vi "HFRR ADV v037 new software.vi"() -> ()   [LabVIEW 2025] (continued)
        n1886 = case shown="True" w2900 {
          frame False {
          }
          frame True {
            n1887 = local write "stopT"(FALSE) -> ()
          }
        }
      }
      frame True {
        "stopT" <- TRUE
      }
    }
    n1888 = case shown="False" w2210 {
      frame False {
      }
      frame True {
      }
    }
    n1889 = case shown="True" w2202 {
      frame False {
        n1890 = property on="Password 2" class="Str"("Visible"=FALSE) -> ()  [unwired: 2 in, 2 out]
        n1891 = local write "Password 2"("" ("Password")) -> ()
      }
      frame True {
        n1892 = property on="Password 2" class="Str"("Visible"=TRUE) -> ()  [unwired: 2 in, 2 out]
        n1893 = Equal?(x="Password 2", y="HFRR1234") -> (x = y?=w2225:bool)
        n1894 = case shown="True" w2225 {
          tunnel: "Password 2" -> [w2228 _]
          frame False {
            n1895 = String Length(string=w2228) -> (length=w2229:i32)
            n1896 = Greater Than 0?(x=w2229) -> (x > 0?=w2227:bool)
            n1897 = case shown="False" w2227 {
              frame False {
                n1898 = property on="Password 2" class="Str"("Caption.Text"="Password (Advance Setting)") -> ()  [unwired: 2 in, 2 out]
              }
              frame True {
                n1899 = property on="Password 2" class="Str"("Caption.Text"="Incorrect Password!") -> ()  [unwired: 2 in, 2 out]
              }
            }
          }
          frame True {
            n1900 = local write "EDIT 2"(FALSE ("EDIT 2")) -> ()
            n1901 = local write "Password 2"("" ("Password")) -> ()
            n1902 = local write "Main Tab"(T2."Advance" ("Main Tab")) -> ()
            n1903 = local write "Main Dashboard Buttons"(T1."Advance" ("Main Dashboard Buttons")) -> ()
          }
        }
      }
    }
    n1904 = case shown="True" "Prog Uno" {
      frame False {
      }
      frame True {
        n1905 = stacked-sequence {
          frame #0 {
            n1906 = Delete(path (use dialog)=path "C:/LAB-IQ-NXT/UNOCOMPILE.bat" ("working directory")) -> ()  [unwired: 4 in, 3 out]
          }
          frame #1 {
            n1907 = local read "Com Port 1"() -> (w2667:refnum<visa-resource-name>)
            n1908 = Concatenate Strings("cmd.exe /c \"mode " ("command line"), w2667, ":1200,n,8,1\"\n" ("command line")) -> (w2672:string)
            n1909 = Concatenate Strings(w2672, "CD\\\nCD WinDucom\navrdude -C avrdude.conf -v -patmega328p -carduino -P" ("command line"), w2667, " -b115200 -D -Uflash:w:UNO_V20.hex:i\n" ("command line"), "\r") -> (w2674:string)
            "STR" <- w2674
            n1910 = call <vilib>:"Write Characters To File.vi"("append to file? (new file:F)"=FALSE, "character string"=w2674, "file path (dialog if empty)"=path "C:/LAB-IQ/UNOCOMPILE.bat" ("working directory")) -> ()  [unwired: 2 in, 1 out]
          }
          frame #2 {
            n1911 = disable-structure shown="Disabled" {
              frame Disabled {
                w2678 = "cmd.exe  /c \"C:\\LAB-IQ-NXT\\UNOCOMPILE.bat\"" ("string")
                n1912 = local write "Prog Uno"(FALSE ("run minimized? (F)")) -> ()
                n1913 = call <vilib>:"System Exec.vi"("expected output size  (4096)"=u32 65535, "run minimized? (F)"=FALSE, "wait until completion? (T)"=TRUE ("run minimized? (F)"), "working directory"=path "C:/LAB-IQ-NXT", "standard input"=w2678, "command line"=w2678) -> ("error out"=w2677:errorcluster, "standard output"=→"String 42":string)  [unwired: 2 in, 2 out]
                "error out 3" <- w2677
                n1914 = flat-sequence {
                  tunnel: w2677 -> [_]
                  frame #0 {
                  }
                }
              }
              frame Enabled {
              }
            }
          }
        }
      }
    }
    n1915 = case shown="\"ISO 12156\"" "TEST STANDARD" {
      frame "ASTM D6079", Default {
        w2647 = 50.0 ("Hz")
        w2648 = 53.0 ("Set Rh")
        w2650 = 1.0 ("Set Strk")
        w2649 = 60.0 ("Set Temp")
        # "astm hide"
        n1916 = local write "NORMAL LOAD"(200.0 ("NORMAL LOAD")) -> ()
        n1917 = local write "Set Strk"(w2650) -> ()
        n1918 = local write "Set Hz"(w2647) -> ()
        n1919 = local write "Set Temp"(w2649) -> ()
        n1920 = local write "Set Rh"(w2648) -> ()
        n1921 = local write "test time"(75.0 ("test time")) -> ()
        n1922 = local write "Set Stroke:"(w2650) -> ()
        n1923 = local write "Set Humidity:"(w2648) -> ()
        n1924 = local write "Set Frequency:"(w2647) -> ()
        n1925 = local write "Set Temperature:"(w2649) -> ()
        "Test Standard" <- "ASTM D6079" ("Test Standard 2")
      }
      frame "ISO 12156" {
        n1926 = local write "Set Strk"(1.0 ("Set Strk")) -> ()
        n1927 = local write "NORMAL LOAD"(200.0 ("NORMAL LOAD")) -> ()
        n1928 = local write "Set Temp"(60.0 ("Set Temp")) -> ()
        n1929 = local write "test time"(75.0 ("test time")) -> ()
        n1930 = local write "Set Hz"(50.0 ("Hz")) -> ()
        n1931 = local write "Set Rh"(53.0 ("Set Rh")) -> ()
      }
      frame "CEC F-096-A-06" {
        n1932 = local write "Set Strk"(1.0 ("Set Strk")) -> ()
        n1933 = local write "NORMAL LOAD"(200.0 ("NORMAL LOAD")) -> ()
        n1934 = local write "Set Temp"(60.0 ("Set Temp")) -> ()
        n1935 = local write "test time"(75.0 ("test time")) -> ()
        n1936 = local write "Set Hz"(50.0 ("Hz")) -> ()
        n1937 = local write "Set Rh"(53.0 ("Set Rh")) -> ()
      }
      frame "Custom" {
      }
    }
    n1938 = Or(x=w2200, y=w2198) -> (x .or. y?=w2199:bool)
    n1939 = case shown="\"About\"" w2197 {
      tunnel: [T28."Acquire" ("Main Tab") T28."Compare Files" ("Main Tab") T28."About" ("Main Tab")] -> w2208
      frame "Acquire", Default {
      }
      frame "Compare Files" {
      }
      frame "About" {
      }
    }
    n1940 = Or(x=w2203, y="OPEN") -> (x .or. y?=w2204:bool)
    n1941 = case shown="True" w2204 {
      tunnel: w2203 -> [_ w2236]
      frame False {
      }
      frame True {
        n1942 = stacked-sequence {
          tunnel: w2236 -> [_ w2303 _ _]
          frame #0 {
            w2252 = "  " ("String 6")
            n1943 = local write "OPEN"(FALSE ("open")) -> ()
            n1944 = local read "string1 2"() -> (w2240:string)
            n1945 = local read "string1 3"() -> (w2239:string)
            n1946 = local read "string1 4"() -> (w2238:string)
            n1947 = property on="OPEN" class="Bool (strict)"("Visible"=FALSE) -> ()  [unwired: 2 in, 2 out]
            n1948 = local write "String 6"(w2252) -> ()
            n1949 = local write "String 7"(w2252) -> ()
            n1950 = local write "String 8"(w2252) -> ()
            n1951 = local write "String 12"(w2252) -> ()
            n1952 = local read "OK Button 16"() -> (w2237:bool)
            n1953 = String To Path(string=w2240) -> (path=w2248:path)
            n1954 = String To Path(string=w2239) -> (path=w2247:path)
            n1955 = String To Path(string=w2238) -> (path=w2246:path)
            n1956 = case shown="True" w2237 {
              tunnel: [w2253 w2254] -> w2241
              frame False {
                n1957 = local read "string1"() -> (w2253:string)
              }
              frame True {
                n1958 = local read "String Indicator 4"() -> (w2254:string)
              }
            }
            n1959 = Open/Create/Replace File "Open File"(file path (use dialog)=w2248) -> (refnum out=w2244:refnum<file>)  [unwired: 5 in, 2 out]
            n1960 = Open/Create/Replace File "Open File"(file path (use dialog)=w2247) -> (refnum out=w2243:refnum<file>)  [unwired: 5 in, 2 out]
            n1961 = Open/Create/Replace File "Open File"(file path (use dialog)=w2246) -> (refnum out=w2242:refnum<file>)  [unwired: 5 in, 2 out]
            n1962 = while {
              tunnel: w2244 -> [w2266]
              i -> [w2262]
              stop <- w2261 continue-if-true
              (unwired) TRUE ("line mode (F)")
              n1963 = Read from Text File "Read File"(file (use dialog)=w2266) -> (text=w2263:string)  [unwired: 3 in, 3 out]
              n1964 = local write "Numeric 11"(w2262) -> ()
              n1965 = String Length(string=w2263) -> (length=w2265:i32)
              n1966 = Greater?(x=w2265, y=1) -> (0:w2261:bool)
            }
            n1967 = while {
              tunnel: w2243 -> [w2272]
              i -> [w2268]
              stop <- w2267 continue-if-true
              (unwired) TRUE ("line mode (F)")
              n1968 = Read from Text File "Read File"(file (use dialog)=w2272) -> (text=w2269:string)  [unwired: 3 in, 3 out]
              n1969 = local write "Numeric 12"(w2268) -> ()
              n1970 = String Length(string=w2269) -> (length=w2271:i32)
              n1971 = Greater?(x=w2271, y=1) -> (0:w2267:bool)
            }
            n1972 = while {
              tunnel: w2242 -> [w2278]
              i -> [w2274]
              stop <- w2273 continue-if-true
              (unwired) TRUE ("line mode (F)")
              n1973 = Read from Text File "Read File"(file (use dialog)=w2278) -> (text=w2275:string)  [unwired: 3 in, 3 out]
              n1974 = local write "Numeric 13"(w2274) -> ()
              n1975 = String Length(string=w2275) -> (length=w2277:i32)
              n1976 = Greater?(x=w2277, y=1) -> (0:w2273:bool)
            }
            n1977 = String To Path(string=w2241) -> (path=w2249:path)
            n1978 = Open/Create/Replace File "Open File"(file path (use dialog)=w2249) -> (refnum out=w2245:refnum<file>)  [unwired: 5 in, 2 out]
            n1979 = while {
              tunnel: w2245 -> [w2260]
              i -> [w2256]
              stop <- w2255 continue-if-true
              (unwired) TRUE ("line mode (F)")
              n1980 = Read from Text File "Read File"(file (use dialog)=w2260) -> (text=w2257:string)  [unwired: 3 in, 3 out]
              n1981 = local write "Numeric 8"(w2256) -> ()
              n1982 = String Length(string=w2257) -> (length=w2259:i32)
              n1983 = Greater?(x=w2259, y=1) -> (0:w2255:bool)
            }
          }
          frame #1 {
            w2430 = FALSE ("ACTUAL   MERGE")
            # "Sample Temp"
            # "ECR"
            # "COF"
            # "Time\nCOF\nFF\nTemp"
            n1984 = case shown="True" w2303 {
              tunnel: [w2450 w2451] -> w2304
              frame False {
                n1985 = local read "string1"() -> (w2450:string)
              }
              frame True {
                n1986 = local read "String Indicator 4"() -> (w2451:string)
              }
            }
            n1987 = local read "string1 3"() -> (w2348:string)
            n1988 = String To Path(string=w2304) -> (path=w2435:path)
            n1989 = String To Path(string=w2348) -> (path=w2446:path)
            n1990 = local read "Numeric 12"() -> (w2432:i32)
            n1991 = local read "Numeric 8"() -> (w2434:i32)
            n1992 = local read "string1 2"() -> (w2349:string)
            n1993 = local read "string1 4"() -> (w2347:string)
            n1994 = Open/Create/Replace File "Open File"(file path (use dialog)=w2435) -> (refnum out=w2449:refnum<file>, error out=w2448:errorcluster)  [unwired: 5 in, 1 out]
            n1995 = Open/Create/Replace File "Open File"(file path (use dialog)=w2446) -> (refnum out=w2442:refnum<file>, error out=w2443:errorcluster)  [unwired: 5 in, 1 out]
            n1996 = for {
              N: w2434 -> [_]
              tunnel: w2449 -> [w2597]
              tunnel: w2448 -> [w2596]
              tunnel: [w2586] -> w2361 mode=indexing
              tunnel: [w2584] -> w2418 mode=indexing
              tunnel: [w2585] -> w2413 mode=indexing
              tunnel: w2430 -> [_]
              tunnel: [w2578] -> w2415 mode=indexing
              tunnel: [w2574] -> w2384 mode=indexing
              tunnel: [w2570] -> w2359 mode=indexing
              tunnel: [w2566] -> w2340 mode=indexing
              tunnel: [w2561] -> w2300 mode=indexing
              (unwired) TRUE ("line mode (F)")
              # "freq"
              # "Stroke"
              # "Time"
              # "CoF"
              # "Humidity"
              # "Temp"
              # "Air Temp"
              # "ECR"
              n1997 = Read from Text File "Read File"(file (use dialog)=w2597, error in=w2596) -> (text=w2562:string)  [unwired: 2 in, 3 out]
              n1998 = local write "String 6"(w2562) -> ()
              n1999 = String Subset(string=w2562, offset (0)=0, length (rest)=14 ("length (rest)")) -> (substring=w2590:string)
              n2000 = String Subset(string=w2562, offset (0)=35, length (rest)=9 ("length (rest)")) -> (substring=w2587:string)
              n2001 = String Subset(string=w2562, offset (0)=15, length (rest)=9 ("length (rest)")) -> (substring=w2593:string)
              n2002 = Fract/Exp String To Number(string=w2590) -> (number=w2586:dbl)  [unwired: 3 in, 1 out]
              n2003 = Fract/Exp String To Number(string=w2587) -> (number=w2585:dbl)  [unwired: 3 in, 1 out]
              n2004 = Fract/Exp String To Number(string=w2593) -> (number=w2584:dbl)  [unwired: 3 in, 1 out]
              n2005 = String Subset(string=w2562, offset (0)=85, length (rest)=9 ("length (rest)")) -> (substring=w2563:string)
              n2006 = String Subset(string=w2562, offset (0)=25, length (rest)=9 ("length (rest)")) -> (substring=w2569:string)
              n2007 = String Subset(string=w2562, offset (0)=55, length (rest)=9 ("length (rest)")) -> (substring=w2571:string)
              n2008 = String Subset(string=w2562, offset (0)=45, length (rest)=9 ("length (rest)")) -> (substring=w2577:string)
              n2009 = String Subset(string=w2562, offset (0)=65, length (rest)=9 ("length (rest)")) -> (substring=w2583:string)
              n2010 = Fract/Exp String To Number(string=w2569) -> (number=w2566:dbl)  [unwired: 3 in, 1 out]
              n2011 = Fract/Exp String To Number(string=w2563) -> (number=w2561:dbl)  [unwired: 3 in, 1 out]
              n2012 = Fract/Exp String To Number(string=w2571) -> (number=w2570:dbl)  [unwired: 3 in, 1 out]
              n2013 = Fract/Exp String To Number(string=w2577) -> (number=w2574:dbl)  [unwired: 3 in, 1 out]
              n2014 = Fract/Exp String To Number(string=w2583) -> (number=w2580:dbl)  [unwired: 3 in, 1 out]
              n2015 = Add(x=w2580, y=0.0) -> (x+y=w2578:dbl)
            }
            n2016 = for {
              N: w2432 -> [_]
              tunnel: w2443 -> [w2523]
              tunnel: w2442 -> [w2522]
              tunnel: [w2512] -> w2401 mode=indexing
              tunnel: [w2510] -> w2399 mode=indexing
              tunnel: [w2511] -> w2395 mode=indexing
              tunnel: w2430 -> [_]
              tunnel: [w2504] -> w2397 mode=indexing
              tunnel: [w2500] -> w2379 mode=indexing
              tunnel: [w2496] -> w2355 mode=indexing
              tunnel: [w2493] -> w2336 mode=indexing
              tunnel: [w2489] -> w2295 mode=indexing
              (unwired) 9 ("length (rest)")
              (unwired) 9 ("length (rest)")
              (unwired) TRUE ("line mode (F)")
              n2017 = Read from Text File "Read File"(file (use dialog)=w2522, error in=w2523) -> (text=w2490:string)  [unwired: 2 in, 3 out]
              n2018 = local write "String 8"(w2490) -> ()
              n2019 = String Subset(string=w2490, offset (0)=85) -> (substring=w2492:string)  [unwired: 1 in]
              n2020 = String Subset(string=w2490, offset (0)=35, length (rest)=9 ("length (rest)")) -> (substring=w2513:string)
              n2021 = String Subset(string=w2490, offset (0)=55, length (rest)=9 ("length (rest)")) -> (substring=w2498:string)
              n2022 = String Subset(string=w2490, offset (0)=25) -> (substring=w2494:string)  [unwired: 1 in]
              n2023 = String Subset(string=w2490, offset (0)=15, length (rest)=9 ("length (rest)")) -> (substring=w2519:string)
              n2024 = String Subset(string=w2490, offset (0)=0, length (rest)=14 ("length (rest)")) -> (substring=w2516:string)
              n2025 = String Subset(string=w2490, offset (0)=45, length (rest)=9 ("length (rest)")) -> (substring=w2503:string)
              n2026 = String Subset(string=w2490, offset (0)=65, length (rest)=9 ("length (rest)")) -> (substring=w2509:string)
              n2027 = Fract/Exp String To Number(string=w2492) -> (number=w2489:dbl)  [unwired: 3 in, 1 out]
              n2028 = Fract/Exp String To Number(string=w2513) -> (number=w2511:dbl)  [unwired: 3 in, 1 out]
              n2029 = Fract/Exp String To Number(string=w2498) -> (number=w2496:dbl)  [unwired: 3 in, 1 out]
              n2030 = Fract/Exp String To Number(string=w2494) -> (number=w2493:dbl)  [unwired: 3 in, 1 out]
              n2031 = Fract/Exp String To Number(string=w2519) -> (number=w2510:dbl)  [unwired: 3 in, 1 out]
              n2032 = Fract/Exp String To Number(string=w2516) -> (number=w2512:dbl)  [unwired: 3 in, 1 out]
              n2033 = Fract/Exp String To Number(string=w2503) -> (number=w2500:dbl)  [unwired: 3 in, 1 out]
              n2034 = Fract/Exp String To Number(string=w2509) -> (number=w2506:dbl)  [unwired: 3 in, 1 out]
              n2035 = Add(x=w2506, y=0.0) -> (x+y=w2504:dbl)
            }
            n2036 = String To Path(string=w2349) -> (path=w2447:path)
            n2037 = String To Path(string=w2347) -> (path=w2441:path)
            n2038 = local read "Numeric 11"() -> (w2431:i32)
            n2039 = local read "Numeric 13"() -> (w2433:i32)
            n2040 = Open/Create/Replace File "Open File"(file path (use dialog)=w2447) -> (refnum out=w2445:refnum<file>, error out=w2444:errorcluster)  [unwired: 5 in, 1 out]
            n2041 = Open/Create/Replace File "Open File"(file path (use dialog)=w2441) -> (refnum out=w2440:refnum<file>, error out=w2439:errorcluster)  [unwired: 5 in, 1 out]
            n2042 = for {
              N: w2431 -> [_]
              tunnel: w2445 -> [w2560]
              tunnel: w2444 -> [w2559]
              tunnel: [w2549] -> w2411 mode=indexing
              tunnel: [w2547] -> w2409 mode=indexing
              tunnel: [w2548] -> w2404 mode=indexing
              tunnel: w2430 -> [_]
              tunnel: [w2541] -> w2406 mode=indexing
              tunnel: [w2537] -> w2382 mode=indexing
              tunnel: [w2533] -> w2357 mode=indexing
              tunnel: [w2529] -> w2338 mode=indexing
              tunnel: [w2524] -> w2296 mode=indexing
              (unwired) TRUE ("line mode (F)")
              n2043 = Read from Text File "Read File"(file (use dialog)=w2560, error in=w2559) -> (text=w2525:string)  [unwired: 2 in, 3 out]
              n2044 = local write "String 7"(w2525) -> ()
              n2045 = String Subset(string=w2525, offset (0)=85, length (rest)=9 ("length (rest)")) -> (substring=w2528:string)
              n2046 = String Subset(string=w2525, offset (0)=35, length (rest)=9 ("length (rest)")) -> (substring=w2550:string)
              n2047 = String Subset(string=w2525, offset (0)=55, length (rest)=9 ("length (rest)")) -> (substring=w2536:string)
              n2048 = String Subset(string=w2525, offset (0)=25, length (rest)=9 ("length (rest)")) -> (substring=w2530:string)
              n2049 = String Subset(string=w2525, offset (0)=45, length (rest)=9 ("length (rest)")) -> (substring=w2538:string)
              n2050 = String Subset(string=w2525, offset (0)=0, length (rest)=14 ("length (rest)")) -> (substring=w2553:string)
              n2051 = String Subset(string=w2525, offset (0)=15, length (rest)=9 ("length (rest)")) -> (substring=w2556:string)
              n2052 = String Subset(string=w2525, offset (0)=65, length (rest)=9 ("length (rest)")) -> (substring=w2542:string)
              n2053 = Fract/Exp String To Number(string=w2528) -> (number=w2524:dbl)  [unwired: 3 in, 1 out]
              n2054 = Fract/Exp String To Number(string=w2550) -> (number=w2548:dbl)  [unwired: 3 in, 1 out]
              n2055 = Fract/Exp String To Number(string=w2536) -> (number=w2533:dbl)  [unwired: 3 in, 1 out]
              n2056 = Fract/Exp String To Number(string=w2530) -> (number=w2529:dbl)  [unwired: 3 in, 1 out]
              n2057 = Fract/Exp String To Number(string=w2538) -> (number=w2537:dbl)  [unwired: 3 in, 1 out]
              n2058 = Fract/Exp String To Number(string=w2553) -> (number=w2549:dbl)  [unwired: 3 in, 1 out]
              n2059 = Fract/Exp String To Number(string=w2556) -> (number=w2547:dbl)  [unwired: 3 in, 1 out]
              n2060 = Fract/Exp String To Number(string=w2542) -> (number=w2545:dbl)  [unwired: 3 in, 1 out]
              n2061 = Add(x=w2545, y=0.0) -> (x+y=w2541:dbl)
            }
            n2062 = for {
              N: w2433 -> [_]
              tunnel: w2440 -> [w2488]
              tunnel: w2439 -> [w2487]
              tunnel: [w2477] -> w2393 mode=indexing
              tunnel: [w2476] -> w2386 mode=indexing
              tunnel: w2430 -> [_]
              tunnel: [w2465] -> w2391 mode=indexing
              tunnel: [w2470] -> w2388 mode=indexing
              tunnel: [w2466] -> w2378 mode=indexing
              tunnel: [w2461] -> w2353 mode=indexing
              tunnel: [w2457] -> w2334 mode=indexing
              tunnel: [w2452] -> w2294 mode=indexing
              (unwired) 1.0 ("x")
              (unwired) TRUE ("line mode (F)")
              n2063 = Read from Text File "Read File"(file (use dialog)=w2488, error in=w2487) -> (text=w2453:string)  [unwired: 2 in, 3 out]
              n2064 = local write "String 12"(w2453) -> ()
              n2065 = String Subset(string=w2453, offset (0)=85, length (rest)=9 ("length (rest)")) -> (substring=w2455:string)
              n2066 = String Subset(string=w2453, offset (0)=35, length (rest)=9 ("length (rest)")) -> (substring=w2478:string)
              n2067 = String Subset(string=w2453, offset (0)=55, length (rest)=9 ("length (rest)")) -> (substring=w2463:string)
              n2068 = String Subset(string=w2453, offset (0)=25, length (rest)=9 ("length (rest)")) -> (substring=w2459:string)
              n2069 = String Subset(string=w2453, offset (0)=45, length (rest)=9 ("length (rest)")) -> (substring=w2468:string)
              n2070 = String Subset(string=w2453, offset (0)=15, length (rest)=9 ("length (rest)")) -> (substring=w2484:string)
              n2071 = String Subset(string=w2453, offset (0)=0, length (rest)=14 ("length (rest)")) -> (substring=w2481:string)
              n2072 = String Subset(string=w2453, offset (0)=65, length (rest)=9 ("length (rest)")) -> (substring=w2471:string)
              n2073 = Fract/Exp String To Number(string=w2455) -> (number=w2452:dbl)  [unwired: 3 in, 1 out]
              n2074 = Fract/Exp String To Number(string=w2478) -> (number=w2476:dbl)  [unwired: 3 in, 1 out]
              n2075 = Fract/Exp String To Number(string=w2463) -> (number=w2461:dbl)  [unwired: 3 in, 1 out]
              n2076 = Fract/Exp String To Number(string=w2459) -> (number=w2457:dbl)  [unwired: 3 in, 1 out]
              n2077 = Fract/Exp String To Number(string=w2468) -> (number=w2466:dbl)  [unwired: 3 in, 1 out]
              n2078 = Fract/Exp String To Number(string=w2484) -> (number=w2465:dbl)  [unwired: 3 in, 1 out]
              n2079 = Fract/Exp String To Number(string=w2481) -> (number=w2477:dbl)  [unwired: 3 in, 1 out]
              n2080 = Fract/Exp String To Number(string=w2471) -> (number=w2474:dbl)  [unwired: 3 in, 1 out]
              n2081 = Add(x=w2474, y=0.0) -> (x+y=w2470:dbl)
            }
            n2082 = Delete From Array(array=w2336, index=0) -> (array with subset deleted=w2309:dbl[])  [unwired: 1 in, 1 out]
            n2083 = Delete From Array(array=w2399, index=0) -> (array with subset deleted=w2372:dbl[])  [unwired: 1 in, 1 out]
            n2084 = Delete From Array(array=w2379, index=0) -> (array with subset deleted=w2367:dbl[])  [unwired: 1 in, 1 out]
            n2085 = Delete From Array(array=w2397, index=0) -> (array with subset deleted=w2398:dbl[])  [unwired: 1 in, 1 out]
            n2086 = call-poly <vilib>:"Mean.vi"("X"=w2309) -> ("mean"=→"КОФ2 4":dbl)  [unwired: 1 out]
            n2087 = call-poly <vilib>:"Mean.vi"("X"=w2372) -> ("mean"=→"КОФ3":dbl)  [unwired: 1 out]
            n2088 = call-poly <vilib>:"Mean.vi"("X"=w2367) -> ("mean"=→"CP3":dbl)  [unwired: 1 out]
            n2089 = Delete From Array(array=w2361, index=0) -> (array with subset deleted=w2288:dbl[])  [unwired: 1 in, 1 out]
            n2090 = Delete From Array(array=w2300, index=0) -> (array with subset deleted=w2287:dbl[])  [unwired: 1 in, 1 out]
            n2091 = Delete From Array(array=w2340, index=0) -> (array with subset deleted=w2311:dbl[])  [unwired: 1 in, 1 out]
            n2092 = Delete From Array(array=w2418, index=0) -> (array with subset deleted=w2373:dbl[])  [unwired: 1 in, 1 out]
            n2093 = Delete From Array(array=w2384, index=0) -> (array with subset deleted=w2369:dbl[])  [unwired: 1 in, 1 out]
            "array w/ subset deleted" <- w2369
            n2094 = Delete From Array(array=w2415, index=0) -> (array with subset deleted=w2416:dbl[])  [unwired: 1 in, 1 out]
            n2095 = call-poly <vilib>:"Mean.vi"("X"=w2311) -> ("mean"=→"КОФ2 2":dbl)  [unwired: 1 out]
            n2096 = call-poly <vilib>:"Mean.vi"("X"=w2373) -> ("mean"=→"КОФ1":dbl)  [unwired: 1 out]
            n2097 = Bundle "Bundle"(w2288, w2287) -> (w2293:cluster{dbl[], dbl[]})  [unwired: 1 in]
            n2098 = Bundle "Bundle"(w2288, w2416) -> (w2280:cluster{dbl[], dbl[]})  [unwired: 1 in]
            n2099 = Delete From Array(array=w2295, index=0) -> (array with subset deleted=w2283:dbl[])  [unwired: 1 in, 1 out]
            n2100 = Delete From Array(array=w2296, index=0) -> (array with subset deleted=w2285:dbl[])  [unwired: 1 in, 1 out]
            n2101 = Delete From Array(array=w2406, index=0) -> (array with subset deleted=w2407:dbl[])  [unwired: 1 in, 1 out]
            n2102 = Delete From Array(array=w2294, index=0) -> (array with subset deleted=w2281:dbl[])  [unwired: 1 in, 1 out]
            n2103 = Delete From Array(array=w2388, index=0) -> (array with subset deleted=w2389:dbl[])  [unwired: 1 in, 1 out]
            n2104 = Delete From Array(array=w2413, index=0) -> (array with subset deleted=w2319:dbl[])  [unwired: 1 in, 1 out]
            n2105 = Delete From Array(array=w2359, index=0) -> (array with subset deleted=w2315:dbl[])  [unwired: 1 in, 1 out]
            n2106 = Delete From Array(array=w2395, index=0) -> (array with subset deleted=w2317:dbl[])  [unwired: 1 in, 1 out]
            n2107 = Delete From Array(array=w2355, index=0) -> (array with subset deleted=w2313:dbl[])  [unwired: 1 in, 1 out]
            n2108 = Delete From Array(array=w2404, index=0) -> (array with subset deleted=w2318:dbl[])  [unwired: 1 in, 1 out]
            n2109 = Delete From Array(array=w2357, index=0) -> (array with subset deleted=w2314:dbl[])  [unwired: 1 in, 1 out]
            n2110 = Delete From Array(array=w2338, index=0) -> (array with subset deleted=w2310:dbl[])  [unwired: 1 in, 1 out]
            n2111 = Delete From Array(array=w2382, index=0) -> (array with subset deleted=w2368:dbl[])  [unwired: 1 in, 1 out]
            n2112 = Delete From Array(array=w2409, index=0) -> (array with subset deleted=w2370:dbl[])  [unwired: 1 in, 1 out]
            n2113 = Delete From Array(array=w2386, index=0) -> (array with subset deleted=w2316:dbl[])  [unwired: 1 in, 1 out]
            n2114 = Delete From Array(array=w2353, index=0) -> (array with subset deleted=w2312:dbl[])  [unwired: 1 in, 1 out]
            n2115 = Delete From Array(array=w2334, index=0) -> (array with subset deleted=w2308:dbl[])  [unwired: 1 in, 1 out]
            n2116 = Delete From Array(array=w2378, index=0) -> (array with subset deleted=w2366:dbl[])  [unwired: 1 in, 1 out]
            n2117 = Delete From Array(array=w2391, index=0) -> (array with subset deleted=w2371:dbl[])  [unwired: 1 in, 1 out]
            n2118 = Delete From Array(array=w2401, index=0) -> (array with subset deleted=w2284:dbl[])  [unwired: 1 in, 1 out]
            n2119 = Delete From Array(array=w2411, index=0) -> (array with subset deleted=w2286:dbl[])  [unwired: 1 in, 1 out]
            n2120 = Delete From Array(array=w2393, index=0) -> (array with subset deleted=w2282:dbl[])  [unwired: 1 in, 1 out]
            n2121 = Bundle "Bundle"(w2288, w2319) -> (w2306:cluster{dbl[], dbl[]})  [unwired: 1 in]
            n2122 = Bundle "Bundle"(w2288, w2373) -> (w2307:cluster{dbl[], dbl[]})  [unwired: 1 in]
            n2123 = Bundle "Bundle"(w2319, w2315) -> (w2321:cluster{dbl[], dbl[]})  [unwired: 1 in]
            n2124 = Bundle "Bundle"(w2284, w2283) -> (w2291:cluster{dbl[], dbl[]})  [unwired: 1 in]
            n2125 = Bundle "Bundle"(w2317, w2313) -> (w2323:cluster{dbl[], dbl[]})  [unwired: 1 in]
            n2126 = Bundle "Bundle"(w2284, w2317) -> (w2427:cluster{dbl[], dbl[]})  [unwired: 1 in]
            n2127 = Bundle "Bundle"(w2284, w2313) -> (w2351:cluster{dbl[], dbl[]})  [unwired: 1 in]
            n2128 = Bundle "Bundle"(w2284, w2372) -> (w2437:cluster{dbl[], dbl[]})  [unwired: 1 in]
            n2129 = Bundle "Bundle"(w2284, w2367) -> (w2375:cluster{dbl[], dbl[]})  [unwired: 1 in]
            n2130 = Bundle "Bundle"(w2284, w2398) -> (w2422:cluster{dbl[], dbl[]})  [unwired: 1 in]
            n2131 = Bundle "Bundle"(w2318, w2314) -> (w2322:cluster{dbl[], dbl[]})  [unwired: 1 in]
            n2132 = Bundle "Bundle"(w2286, w2285) -> (w2292:cluster{dbl[], dbl[]})  [unwired: 1 in]
            n2133 = Bundle "Bundle"(w2286, w2318) -> (w2429:cluster{dbl[], dbl[]})  [unwired: 1 in]
            n2134 = Bundle "Bundle"(w2286, w2314) -> (w2352:cluster{dbl[], dbl[]})  [unwired: 1 in]
            n2135 = Bundle "Bundle"(w2286, w2368) -> (w2376:cluster{dbl[], dbl[]})  [unwired: 1 in]
            n2136 = Bundle "Bundle"(w2286, w2370) -> (w2438:cluster{dbl[], dbl[]})  [unwired: 1 in]
            n2137 = Bundle "Bundle"(w2286, w2407) -> (w2420:cluster{dbl[], dbl[]})  [unwired: 1 in]
            n2138 = Bundle "Bundle"(w2316, w2312) -> (w2324:cluster{dbl[], dbl[]})  [unwired: 1 in]
            n2139 = Bundle "Bundle"(w2282, w2281) -> (w2290:cluster{dbl[], dbl[]})  [unwired: 1 in]
            n2140 = Bundle "Bundle"(w2282, w2316) -> (w2428:cluster{dbl[], dbl[]})  [unwired: 1 in]
            n2141 = Bundle "Bundle"(w2282, w2312) -> (w2350:cluster{dbl[], dbl[]})  [unwired: 1 in]
            n2142 = Bundle "Bundle"(w2282, w2366) -> (w2374:cluster{dbl[], dbl[]})  [unwired: 1 in]
            n2143 = Bundle "Bundle"(w2282, w2371) -> (w2436:cluster{dbl[], dbl[]})  [unwired: 1 in]
            n2144 = Bundle "Bundle"(w2282, w2389) -> (w2421:cluster{dbl[], dbl[]})  [unwired: 1 in]
            n2145 = call-poly <vilib>:"Mean.vi"("X"=w2369) -> ("mean"=→"CP1":dbl)  [unwired: 1 out]
            n2146 = call-poly <vilib>:"Mean.vi"("X"=w2310) -> ("mean"=→"КОФ2 3":dbl)  [unwired: 1 out]
            n2147 = call-poly <vilib>:"Mean.vi"("X"=w2368) -> ("mean"=→"CP2":dbl)  [unwired: 1 out]
            n2148 = call-poly <vilib>:"Mean.vi"("X"=w2370) -> ("mean"=→"КОФ2":dbl)  [unwired: 1 out]
            n2149 = call-poly <vilib>:"Mean.vi"("X"=w2308) -> ("mean"=→"КОФ2 5":dbl)  [unwired: 1 out]
            n2150 = call-poly <vilib>:"Mean.vi"("X"=w2366) -> ("mean"=→"CP4":dbl)  [unwired: 1 out]
            n2151 = call-poly <vilib>:"Mean.vi"("X"=w2371) -> ("mean"=→"КОФ4":dbl)  [unwired: 1 out]
            n2152 = Bundle "Bundle"(w2288, w2315) -> (w2279:cluster{dbl[], dbl[]})  [unwired: 1 in]
            n2153 = Bundle "Bundle"(w2288, w2369) -> (w2302:cluster{dbl[], dbl[]})  [unwired: 1 in]
            n2154 = Build Array "Build Array"(w2279, w2302) -> (w2305:cluster{dbl[], dbl[]}[])
            "XY Graph 17" <- w2305
            n2155 = Build Array "Build Array"(w2293, w2292, w2291, w2290) -> (→"Frequency ( Hz )":cluster{dbl[], dbl[]}[])
            n2156 = Build Array "Build Array"(w2321, w2322, w2323, w2324) -> (→"Air Temp ( °C ) vs Humidity ( % RH )":cluster{dbl[], dbl[]}[])
            n2157 = Build Array "Build Array"(w2306, w2429, w2427, w2428) -> (→"Air Temperature  ( °C )":cluster{dbl[], dbl[]}[])
            n2158 = Build Array "Build Array"(w2279, w2352, w2351, w2350) -> (→"Humidity ( %RH )":cluster{dbl[], dbl[]}[])
            n2159 = Build Array "Build Array"(w2307, w2438, w2437, w2436) -> (→"Coefficient Of Friction":cluster{dbl[], dbl[]}[])
            n2160 = Build Array "Build Array"(w2302, w2376, w2375, w2374) -> (→"Sample Temperature ( °C )":cluster{dbl[], dbl[]}[])
            n2161 = Build Array "Build Array"(w2280, w2420, w2422, w2421) -> (→"XY Graph 13":cluster{dbl[], dbl[]}[])
            n2162 = Bundle "Bundle"(w2288, w2311) -> (w2333:cluster{dbl[], dbl[]})  [unwired: 1 in]
            n2163 = Bundle "Bundle"(w2284, w2309) -> (w2331:cluster{dbl[], dbl[]})  [unwired: 1 in]
            n2164 = Bundle "Bundle"(w2286, w2310) -> (w2332:cluster{dbl[], dbl[]})  [unwired: 1 in]
            n2165 = Bundle "Bundle"(w2282, w2308) -> (w2330:cluster{dbl[], dbl[]})  [unwired: 1 in]
            n2166 = Build Array "Build Array"(w2333, w2332, w2331, w2330) -> (→"Stroke ( mm )":cluster{dbl[], dbl[]}[])
            n2167 = local write "XY Graph 16"(w2305) -> ()
          }
          frame #2 {
          }
          frame #3 {
            n2168 = local write "Numeric 8"(0 ("Numeric 8")) -> ()
            n2169 = local write "Numeric 11"(0 ("Numeric 11")) -> ()
            n2170 = local write "Numeric 12"(0 ("Numeric 12")) -> ()
            n2171 = local write "Numeric 13"(0 ("Numeric 13")) -> ()
            n2172 = property on="OPEN" class="Bool (strict)"("Visible"=TRUE) -> ()  [unwired: 2 in, 2 out]
            n2173 = local read "String Control 2"() -> (w2605:string)
            n2174 = local read "String Control 4"() -> (w2604:string)
            n2175 = local read "String Control 6"() -> (w2603:string)
            n2176 = local read "String Control 8"() -> (w2602:string)
            n2177 = Match Pattern(string=w2605, regular expression="Samples / cycle :- ") -> (after substring=w2619:string)  [unwired: 1 in, 3 out]
            n2178 = Match Pattern(string=w2605, regular expression="Frequency :- ") -> (after substring=w2638:string)  [unwired: 1 in, 3 out]
            n2179 = Match Pattern(string=w2604, regular expression="Samples / cycle :- ") -> (after substring=w2615:string)  [unwired: 1 in, 3 out]
            n2180 = Match Pattern(string=w2604, regular expression="Frequency :- ") -> (after substring=w2633:string)  [unwired: 1 in, 3 out]
            n2181 = Match Pattern(string=w2603, regular expression="Samples / cycle :- ") -> (after substring=w2611:string)  [unwired: 1 in, 3 out]
            n2182 = Match Pattern(string=w2603, regular expression="Frequency :- ") -> (after substring=w2628:string)  [unwired: 1 in, 3 out]
            n2183 = Match Pattern(string=w2602, regular expression="Samples / cycle :- ") -> (after substring=w2607:string)  [unwired: 1 in, 3 out]
            n2184 = Match Pattern(string=w2602, regular expression="Frequency :- ") -> (after substring=w2623:string)  [unwired: 1 in, 3 out]
            n2185 = String Subset(string=w2619, length (rest)=6 ("length (rest)")) -> (substring=w2621:string)  [unwired: 1 in]
            n2186 = String Subset(string=w2638, length (rest)=9 ("length (rest)")) -> (substring=w2640:string)  [unwired: 1 in]
            n2187 = String Subset(string=w2615, length (rest)=6 ("length (rest)")) -> (substring=w2617:string)  [unwired: 1 in]
            n2188 = String Subset(string=w2633, length (rest)=9 ("length (rest)")) -> (substring=w2635:string)  [unwired: 1 in]
            n2189 = String Subset(string=w2611, length (rest)=6 ("length (rest)")) -> (substring=w2613:string)  [unwired: 1 in]
            n2190 = String Subset(string=w2628, length (rest)=9 ("length (rest)")) -> (substring=w2630:string)  [unwired: 1 in]
            n2191 = String Subset(string=w2607, length (rest)=6 ("length (rest)")) -> (substring=w2609:string)  [unwired: 1 in]
            n2192 = String Subset(string=w2623, length (rest)=9 ("length (rest)")) -> (substring=w2625:string)  [unwired: 1 in]
            n2193 = Fract/Exp String To Number(string=w2621) -> (number=w2601:dbl)  [unwired: 3 in, 1 out]
            n2194 = Fract/Exp String To Number(string=w2640) -> (number=w2641:dbl)  [unwired: 3 in, 1 out]
            n2195 = Fract/Exp String To Number(string=w2617) -> (number=w2600:dbl)  [unwired: 3 in, 1 out]
            n2196 = Fract/Exp String To Number(string=w2635) -> (number=w2636:dbl)  [unwired: 3 in, 1 out]
            n2197 = Fract/Exp String To Number(string=w2613) -> (number=w2599:dbl)  [unwired: 3 in, 1 out]
            n2198 = Fract/Exp String To Number(string=w2630) -> (number=w2631:dbl)  [unwired: 3 in, 1 out]
            n2199 = Fract/Exp String To Number(string=w2609) -> (number=w2598:dbl)  [unwired: 3 in, 1 out]
            n2200 = Fract/Exp String To Number(string=w2625) -> (number=w2626:dbl)  [unwired: 3 in, 1 out]
            n2201 = local write "sample1"(w2601) -> ()
            n2202 = local write "freq1"(w2641) -> ()
            n2203 = local write "sample2"(w2600) -> ()
            n2204 = local write "freq2"(w2636) -> ()
            n2205 = local write "sample3"(w2599) -> ()
            n2206 = local write "freq3"(w2631) -> ()
            n2207 = local write "sample4"(w2598) -> ()
            n2208 = local write "freq 4"(w2626) -> ()
          }
        }
      }
    }
    n2209 = case shown="True" w2199 {
      selector: w2199 -> [_ w2218]
      frame False {
      }
      frame True {
        n2210 = Not(x=w2218) -> (.not. x?=w2214:bool)
        n2211 = local write "service 3"(w2214) -> ()
        n2212 = local write "OPEN 6"(w2214) -> ()
        n2213 = call <vilib>:"System Exec.vi"("wait until completion? (T)"=TRUE, "command line"="C:\\LAB-IQ\\Scar View.exe") -> ("error out"=→"error out 5":errorcluster)  [unwired: 6 in, 3 out]
      }
    }
    n2214 = case shown="\"Acquire\", Default" w2208 {
      frame "Acquire", Default {
        # "Elapsed time\ncof\nstroke\nAir temp\nTemp\nHumidity"
        n2215 = disable-structure shown="Disabled" {
          frame Disabled {
            n2216 = local read "Flag"() -> (w2917:dbl)
            n2217 = local read "RUN"() -> (w2914:bool)
            n2218 = Not(x=w2914) -> (.not. x?=w2913:bool)
            n2219 = Equal?(x=w2917, y=10.0) -> (x = y?=w2915:bool)
            n2220 = And(x=w2915, y=w2913) -> (x .and. y?=w2912:bool)
            n2221 = case shown="True" w2912 {
              frame False {
              }
              frame True {
                w2918 = FALSE ("Heater Button")
                n2222 = local write "Humidity"(w2918) -> ()
                n2223 = local write "Heater Button"(w2918) -> ()
              }
            }
          }
          frame Enabled {
          }
        }
        n2224 = disable-structure shown="Disabled" {
          frame Disabled {
            n2225 = case shown="True" {
              selector: _ -> [_ _]
              frame False {
              }
              frame True {
                w2967 = TRUE ("Heater")
                n2226 = local write "Humidity"(w2967) -> ()
                n2227 = local write "Heater Button"(w2967) -> ()
                n2228 = local read "TEST STANDARD"() -> (w2970:T3)
                n2229 = local read "TEST STANDARD"() -> (w2965:T3)
                n2230 = Equal?(x=w2970, y=enum16{"ASTM D6079", "ISO 12156", "Custom"}."ISO 12156" ("Test Standard")) -> (x = y?=w2968:bool)
                n2231 = Equal?(x=w2965, y=enum16{"ASTM D6079", "ISO 12156", "Custom"}."ASTM D6079" ("Test Standard")) -> (x = y?=w2964:bool)
                n2232 = case shown="True" w2968 {
                  frame False {
                  }
                  frame True {
                    n2233 = local write "airtempflg"(FALSE ("airtempflg")) -> ()
                    n2234 = local write item#-1(TRUE ("Heater")) -> ()
                  }
                }
                n2235 = case shown="True" w2964 {
                  frame False {
                  }
                  frame True {
                    n2236 = local write "airtempflg"(TRUE ("airtempflg")) -> ()
                    n2237 = local write item#-1(FALSE ("Heater")) -> ()
                  }
                }
              }
            }
          }
          frame Enabled {
          }
        }
        n2238 = stacked-sequence {
          frame #0 {
            n2239 = case shown="True" "RST FF" {
              frame False {
              }
              frame True {
                w2984 = 0.0 ("X Scale.Range:Maximum")
                n2240 = property on="Frictional Force ( N )" class="WFChart (strict)"("XScale.Maximum"=600.0 ("X Scale.Range:Maximum"), "XScale.Minimum"=w2984, "YScale.Maximum"=10.0 ("Y Scale.Range:Maximum"), "YScale.Minimum"=w2984) -> ()  [unwired: 2 in, 2 out]
              }
            }
          }
          frame #1 {
            n2241 = case shown="True" "RST TEMP" {
              frame False {
              }
              frame True {
                n2242 = property on="Temperature ( Deg C )" class="WFChart (strict)"("XScale.Minimum"=0.0 ("X Scale.Range:Minimum"), "XScale.Maximum"=600.0 ("X Scale.Range:Maximum"), "YScale.Minimum"=0.0 ("Y Scale.Range:Minimum"), "YScale.Maximum"=100.0 ("Y Scale.Range:Maximum")) -> ()  [unwired: 2 in, 2 out]
              }
            }
          }
          frame #2 {
            n2243 = case shown="True" "RSTCOF" {
              frame False {
              }
              frame True {
                n2244 = property on="Coefficient of Friction" class="WFChart (strict)"("XScale.Minimum"=0.0 ("X Scale.Range:Minimum"), "XScale.Maximum"=600.0 ("X Scale.Range:Maximum"), "YScale.Maximum"=1.0 ("X Scale.Range:Minimum"), "YScale.Minimum"=0.0 ("X Scale.Range:Minimum")) -> ()  [unwired: 2 in, 2 out]
              }
            }
          }
          frame #3 {
            n2245 = case shown="True" "RSTCOF 2" {
              frame False {
              }
              frame True {
                (unwired) 100.0 ("Y Scale.Range:Maximum")
                (unwired) 0.0 ("Y Scale.Range:Minimum")
                (unwired) 600.0 ("X Scale.Range:Maximum")
                (unwired) 0.0 ("X Scale.Range:Minimum")
              }
            }
          }
          frame #4 {
            n2246 = case shown="True" "RSTCOF 3" {
              frame False {
              }
              frame True {
                n2247 = property on="Electrical Contact Resistance ( % )" class="WFChart (strict)"("XScale.Minimum"=0.0 ("X Scale.Range:Minimum"), "XScale.Maximum"=600.0 ("X Scale.Range:Maximum"), "YScale.Minimum"=0.0 ("Y Scale.Range:Minimum"), "YScale.Maximum"=100.0 ("Y Scale.Range:Maximum")) -> ()  [unwired: 2 in, 2 out]
              }
            }
          }
        }
        n2248 = local read "RUN"() -> (w2907:bool)
        n2249 = case shown="False" w2907 {
          frame False {
          }
          frame True {
          }
        }
        n2250 = local read "RUN"() -> (w2911:bool)
        n2251 = case shown="False" w2911 {
          tunnel: [FALSE ("TEST RUNNING") TRUE ("TEST RUNNING")] -> w2910
          frame False {
            w3003 = 0.0 ("Flag")
            n2252 = local write "Elapsed time"(0.0 ("elapsedtime")) -> ()
            n2253 = local write "Time Remaining"(w3003) -> ()
            n2254 = local write "Flag"(w3003) -> ()
            n2255 = local write "Remaining Time"(w3003) -> ()
          }
          frame True {
            n2256 = local write "Flag"(10.0 ("Flag")) -> ()
          }
        }
        n2257 = local read "AIR TEMP"() -> (w2905:dbl)
        n2258 = Greater Or Equal?(x=w2905, y=15.0) -> (x >= y?=w2906:bool)
        "powstat" <- w2906
        n2259 = case shown="True" "Save & Continue" {
          frame False {
          }
          frame True {
            n2260 = local read "USER ID"() -> (w3311:string)
            n2261 = local read "FILE"() -> (w3319:string)
            n2262 = String Length(string=w3319) -> (length=w3317:i32)
            n2263 = String Length(string=w3311) -> (length=w3314:i32)
            n2264 = Greater?(x=w3317, y=0) -> (0:w3316:bool)
            n2265 = Greater?(x=w3314, y=0) -> (0:w3313:bool)
            n2266 = And(x=w3316, y=w3313) -> (x .and. y?=w3312:bool)
            n2267 = case shown="True" w3312 {
              frame False {
                n2268 = stacked-sequence {
                  frame #0 {
                    n2269 = One Button Dialog(message="Please Enter a File Name and Operator ID to save data !", button name ("OK")="Ok") -> ()  [unwired: 1 out]
                  }
                  frame #1 {
                    n2270 = local write "Save & Continue"(FALSE ("OK Button")) -> ()
                  }
                }
                n2271 = local write "Save & Continue"(FALSE ("OK Button")) -> ()
              }
              frame True {
                n2272 = stacked-sequence {
                  frame #0 {
                    n2273 = local read "FILE"() -> (w3325:string)
                    n2274 = call "file check.vi"("file name in"=w3325) -> ("file name out"=w3324:string)  [unwired: 9 in, 1 out]
                    n2275 = call <vilib>:"Application Directory.vi"() -> ("Application Directory"=w3335:path)
                    n2276 = Build Path(base path=w3335, name or relative path="data") -> (appended path=w3334:path)
                    n2277 = call <vilib>:"Trim Whitespace.vi"("string"=w3324) -> ("trimmed string"=w3332:string)  [unwired: 1 in]
                    n2278 = call <vilib>:"Trim Whitespace.vi"("string"=w3324) -> ("trimmed string"=w3333:string)  [unwired: 1 in]
                    n2279 = List Folder(path=w3334) -> (folder names=w3330:string[])  [unwired: 3 in, 3 out]
                    n2280 = Match Pattern(string=w3332, regular expression="_(") -> (before substring=w3329:string)  [unwired: 1 in, 3 out]
                    n2281 = for {
                      tunnel: w3330 -> [w3344] mode=indexing
                      tunnel: w3329 -> [w3342]
                      shift-right: [w3340] -> w3327
                      shift-left: bool[] [] -> [w3341]
                      n2282 = Match Pattern(string=w3344, regular expression="_(") -> (before substring=w3343:string)  [unwired: 1 in, 3 out]
                      n2283 = Equal?(x=w3343, y=w3342) -> (x = y?=w3339:bool)
                      n2284 = case shown="True" w3339 {
                        tunnel: w3339 -> [_ w3347]
                        tunnel: w3341 -> [w3346 w3349]
                        tunnel: [w3346 w3348] -> w3340
                        frame False {
                        }
                        frame True {
                          n2285 = Insert Into Array(array=w3349, new element=w3347) -> (w3348:bool[])  [unwired: 1 in]
                        }
                      }
                    }
                    n2286 = Equal?(x=w3330, y=w3329) -> (x = y?=w3338:bool[])
                    n2287 = Or Array Elements(Boolean array=w3338) -> (logical OR=w3337:bool)
                    n2288 = Array Size(array=w3327) -> (size(s)=w3326:i32)
                    n2289 = case shown="True" w3337 {
                      tunnel: w3333 -> [_ w3357]
                      tunnel: w3326 -> [_ w3350]
                      frame False {
                      }
                      frame True {
                        n2290 = Number To Decimal String(number=w3350) -> (decimal integer string=w3353:string)  [unwired: 1 in]
                        n2291 = Search/Split String(string=w3357, search string/char (-)="_(" ("regular expression")) -> (substring before match=w3355:string)  [unwired: 1 in, 2 out]
                        n2292 = Concatenate Strings(w3355, "_(" ("regular expression"), w3353, ")" ("regular expression")) -> (w3351:string)
                        n2293 = local write "FILE"(w3351) -> ()
                      }
                    }
                  }
                  frame #1 {
                    w3360 = 0.0
                    w3373 = cluster{"y":dbl, dbl, "y":dbl}[] [] ("History Data")
                    w3374 = FALSE ("Heater Button")
                    (unwired) ")!" ("string")
                    (unwired) ")" ("string")
                    w3372 = dbl[] [] ("History Data")
                    w3378 = "\r"
                    # "C:\\WinDucom\\Data\\"
                    # "C:\\LAB-IQ-NXT\\data"
                    n2294 = local write "Humidity ( %RH )"(w3360) -> ()
                    n2295 = local write "Frequency ( Hz )"(w3360) -> ()
                    n2296 = local write "Stroke 3"(w3360) -> ()
                    n2297 = local write "speedop"(0.0 ("PIDclk 2")) -> ()
                    n2298 = local write "Set Temp 2"(65.0 ("Set Temp 2")) -> ()
                    n2299 = local write "AIR TEMP"(w3360) -> ()
                    n2300 = local write "clk"(0.0 ("clk")) -> ()
                    n2301 = local write "Stroke 4"(w3360) -> ()
                    n2302 = local write "COF 2"(w3360) -> ()
                    n2303 = local write "TEMP"(w3360) -> ()
                    n2304 = local write "ecr 3"(w3360) -> ()
                    n2305 = local write "FF 3"(w3360) -> ()
                    n2306 = local write "FF 2"(w3360) -> ()
                    n2307 = property on="Humidity ( %RH ) 2" class="WFChart (strict)"("History Data"=w3372) -> ()  [unwired: 2 in, 2 out]
                    n2308 = property on="Coefficient of Friction" class="WFChart (strict)"("History Data"=w3372) -> ()  [unwired: 2 in, 2 out]
                    n2309 = property on="Coefficient of Friction" class="WFChart (strict)"("History Data"=w3372) -> ()  [unwired: 2 in, 2 out]
                    n2310 = property on="Frictional Force ( N )" class="WFChart (strict)"("History Data"=w3372) -> ()  [unwired: 2 in, 2 out]
                    n2311 = property on="Electrical Contact Resistance ( % )" class="WFChart (strict)"("History Data"=w3372) -> ()  [unwired: 2 in, 2 out]
                    n2312 = property on="Electrical Contact Resistance ( % )" class="WFChart (strict)"("History Data"=w3372) -> ()  [unwired: 2 in, 2 out]
                    n2313 = property on="Temperature ( Deg C )" class="WFChart (strict)"("History Data"=w3372) -> ()  [unwired: 2 in, 2 out]
                    n2314 = property on="Frictional Force ( N )" class="WFChart (strict)"("History Data"=w3372) -> ()  [unwired: 2 in, 2 out]
                    n2315 = property on="Coefficient of Friction" class="WFChart (strict)"("History Data"=w3372) -> ()  [unwired: 2 in, 2 out]
                    n2316 = property on="Frictional Force ( N )" class="WFChart (strict)"("History Data"=w3372) -> ()  [unwired: 2 in, 2 out]
                    n2317 = property on="Electrical Contact Resistance ( % )" class="WFChart (strict)"("History Data"=w3372) -> ()  [unwired: 2 in, 2 out]
                    n2318 = property on="Temperature ( Deg C )" class="WFChart (strict)"("History Data"=w3372) -> ()  [unwired: 2 in, 2 out]
                    n2319 = property on="Stroke ( mm )" class="WFChart (strict)"("History Data"=w3373) -> ()  [unwired: 2 in, 2 out]
                    n2320 = property on="Stroke ( mm )" class="WFChart (strict)"("History Data"=w3373) -> ()  [unwired: 2 in, 2 out]
                    n2321 = local write "Humidity"(w3374) -> ()
                    n2322 = local write "Heater Button"(w3374) -> ()
                    n2323 = local read "FILE"() -> (w3368:string)
                    n2324 = disable-structure shown="Enabled" {
                      disable-tunnel: [w3412 _] -> w3359
                      frame Enabled {
                        n2325 = local read "NORMAL LOAD"() -> (w3412:dbl)
                      }
                      frame Disabled {
                      }
                    }
                    n2326 = call "file check.vi"("file name in"=w3368) -> ("error out"=w3371:errorcluster, "file name out"=w3365:string)  [unwired: 9 in]
                    n2327 = call "FILE PATH CREATION.vi"("error in"=w3371, "FILE NAME :"=w3365) -> ("FILE OUT"=w3364:path)  [unwired: 8 in, 1 out]
                    n2328 = Concatenate Strings(w3365, ".dgf" ("Substring")) -> (w3370:string)
                    n2329 = Concatenate Strings(w3365, ".duf" ("Substring")) -> (w3366:string)
                    n2330 = Multiply(x=w3359, y=1.0) -> (x*y=w3391:dbl)
                    n2331 = Build Path(base path=w3364, name or relative path=w3370) -> (appended path=w3363:path)
                    n2332 = Build Path(base path=w3364, name or relative path=w3366) -> (appended path=w3362:path)
                    n2333 = Number To Fractional String(number=w3391, width (-)=i16 5, precision (6)=i16 2) -> (F-format string=w3399:string)  [unwired: 1 in]
                    n2334 = local read "tested by"() -> (w3358:string)
                    n2335 = local read "Fuel Discription :"() -> (w3387:string)
                    n2336 = local read "Batch Ref Num :"() -> (w3376:string)
                    n2337 = Get Date/Time String(date format (0)=enum16{"short", "long", "abbreviated"}."short") -> (date string=w3410:string, time string=w3407:string)  [unwired: 2 in]
                    n2338 = local read "Remarks :"() -> (w3386:string)
                    n2339 = Concatenate Strings("Load :- " ("Substring"), w3399, " grams ," ("Substring")) -> (w3398:string)
                    n2340 = local read "String 41"() -> (w3379:string)
                    n2341 = Concatenate Strings(w3387) -> (w3388:string)
                    n2342 = Concatenate Strings(w3376) -> (w3375:string)
                    n2343 = Concatenate Strings(w3358) -> (w3382:string)
                    n2344 = Concatenate Strings("(" ("Substring"), w3410, ")" ("Substring"), w3407) -> (w3381:string)
                    "concatenated string" <- w3381
                    n2345 = Concatenate Strings(w3386, "," ("string")) -> (w3385:string)
                    n2346 = Concatenate Strings("  TIME;      COF;       STROKE;     AIR TEMP;  TEMP;  HUMIDITY;  ECR; PID-OUT; FREQUENCY" ("Substring"), "\r") -> (w3394:string)
                    n2347 = Concatenate Strings(w3379, w3378, "Fuel Discription :-" ("Substring"), w3388, w3378, w3398, w3378, "Batch Ref Num :-" ("Substring"), w3375, w3378, " Remarks :- " ("Substring"), w3385, w3378, " Date :- " ("Substring"), w3381, w3378, "Tested By :-" ("Substring"), w3382) -> (w3392:string)
                    "REMARKS" <- w3392
                    n2348 = call <vilib>:"Write Characters To File.vi"("append to file? (new file:F)"=FALSE, "character string"=w3394, "file path (dialog if empty)"=w3363) -> ()  [unwired: 2 in, 1 out]
                    n2349 = call <vilib>:"Write Characters To File.vi"("append to file? (new file:F)"=FALSE, "character string"=w3392, "file path (dialog if empty)"=w3362) -> ()  [unwired: 2 in, 1 out]
                  }
                  frame #2 {
                    n2350 = local write "Cycles elapsed"(0 ("Cycles elapsed")) -> ()
                    n2351 = local write "cyclecount"(0 ("cyclecount")) -> ()
                    n2352 = local write "Save & Continue"(FALSE ("OK")) -> ()
                    n2353 = local write "autostrtflg"(TRUE ("autostrtflg")) -> ()
                    n2354 = local write "Save"(FALSE ("Save")) -> ()
                    n2355 = Get Date/Time In Seconds() -> (seconds since 1Jan1904=w3417:timestamp)
                    n2356 = To Double Precision Float(number=w3417) -> (double precision float=w3416:dbl)
                    n2357 = local write "acq timer"(w3416) -> ()
                    n2358 = One Button Dialog(message="Please ensure sample is mounted properly and machine is ready in all aspects for testing !", button name ("OK")="Ok") -> ()  [unwired: 1 out]
                  }
                  frame #3 {
                    n2359 = stacked-sequence {
                      frame #0 {
                        n2360 = local write "Main Dashboard Buttons"(T1."Dashboard" ("Main Dashboard Buttons")) -> ()
                        n2361 = local write "Main Tab"(T2."Acquire" ("Main Tab")) -> ()
                      }
                      frame #1 {
                        n2362 = local write "EVENT LOG"("" ("EVENT LOG")) -> ()
                      }
                      frame #2 {
                        n2363 = Wait (ms)(milliseconds to wait=u32 50) -> ()  [unwired: 1 out]
                      }
                      frame #3 {
                        n2364 = disable-structure shown="Disabled" {
                          frame Disabled {
                            n2365 = local read "EVENT LOG"() -> (w3429:string)
                            n2366 = call "Event Log.vi"("Content"="Test Details", "EVENT LOG"=w3429) -> ("EVENT LOG"=w3428:string)  [unwired: 8 in, 1 out]
                            n2367 = local write "EVENT LOG"(w3428) -> ()
                          }
                          frame Enabled {
                          }
                        }
                      }
                      frame #4 {
                        n2368 = Wait (ms)(milliseconds to wait=u32 50) -> ()  [unwired: 1 out]
                      }
                      frame #5 {
                        n2369 = local read "FILE"() -> (w3431:string)
                        n2370 = Concatenate Strings("File Name :" ("Content"), w3431) -> (w3432:string)
                        n2371 = local read "EVENT LOG"() -> (w3435:string)
                        n2372 = call "Event Log.vi"("Content"=w3432, "EVENT LOG"=w3435) -> ("EVENT LOG"=w3434:string)  [unwired: 8 in, 1 out]
                        n2373 = local write "EVENT LOG"(w3434) -> ()
                      }
                      frame #6 {
                        n2374 = Wait (ms)(milliseconds to wait=u32 50) -> ()  [unwired: 1 out]
                      }
                      frame #7 {
                        n2375 = local read "Batch Ref Num :"() -> (w3437:string)
                        n2376 = Concatenate Strings("Batch Ref No :" ("Content"), w3437) -> (w3438:string)
                        n2377 = local read "EVENT LOG"() -> (w3441:string)
                        n2378 = call "Event Log.vi"("Content"=w3438, "EVENT LOG"=w3441) -> ("EVENT LOG"=w3440:string)  [unwired: 8 in, 1 out]
                        n2379 = local write "EVENT LOG"(w3440) -> ()
                      }
                      frame #8 {
                        n2380 = Wait (ms)(milliseconds to wait=u32 50) -> ()  [unwired: 1 out]
                      }
                      frame #9 {
                        n2381 = local read "tested by"() -> (w3443:string)
                        n2382 = Concatenate Strings("Tested By :" ("Content"), w3443) -> (w3444:string)
                        n2383 = local read "EVENT LOG"() -> (w3447:string)
                        n2384 = call "Event Log.vi"("Content"=w3444, "EVENT LOG"=w3447) -> ("EVENT LOG"=w3446:string)  [unwired: 8 in, 1 out]
                        n2385 = local write "EVENT LOG"(w3446) -> ()
                      }
                      frame #10 {
                        n2386 = Wait (ms)(milliseconds to wait=u32 50) -> ()  [unwired: 1 out]
                      }
                      frame #11 {
                        n2387 = local read "TEST STANDARD"() -> (w3450:T3)
                        n2388 = case shown="\"ASTM D6079\", Default" w3450 {
                          tunnel: ["ASTM D6079" "ISO 12156" "CEC F-096-A-06" "Custom"] -> w3449
                          frame "ASTM D6079", Default {
                          }
                          frame "ISO 12156" {
                          }
                          frame "CEC F-096-A-06" {
                          }
                          frame "Custom" {
                          }
                        }
                        n2389 = Concatenate Strings("Test Standard :" ("Content"), w3449) -> (w3451:string)
                        n2390 = local read "EVENT LOG"() -> (w3454:string)
                        n2391 = call "Event Log.vi"("Content"=w3451, "EVENT LOG"=w3454) -> ("EVENT LOG"=w3453:string)  [unwired: 8 in, 1 out]
                        n2392 = local write "EVENT LOG"(w3453) -> ()
                      }
                      frame #12 {
                        n2393 = Wait (ms)(milliseconds to wait=u32 50) -> ()  [unwired: 1 out]
                      }
                      frame #13 {
                        n2394 = local read "Fuel Discription :"() -> (w3460:string)
                        n2395 = Concatenate Strings("Fuel Description :" ("Content"), w3460) -> (w3461:string)
                        n2396 = local read "EVENT LOG"() -> (w3464:string)
                        n2397 = call "Event Log.vi"("Content"=w3461, "EVENT LOG"=w3464) -> ("EVENT LOG"=w3463:string)  [unwired: 8 in, 1 out]
                        n2398 = local write "EVENT LOG"(w3463) -> ()
                      }
                      frame #14 {
                        n2399 = Wait (ms)(milliseconds to wait=u32 50) -> ()  [unwired: 1 out]
                      }
                      frame #15 {
                        n2400 = local read "Remarks :"() -> (w3466:string)
                        n2401 = Concatenate Strings("Remarks :" ("Content"), w3466) -> (w3467:string)
                        n2402 = local read "EVENT LOG"() -> (w3470:string)
                        n2403 = call "Event Log.vi"("Content"=w3467, "EVENT LOG"=w3470) -> ("EVENT LOG"=w3469:string)  [unwired: 8 in, 1 out]
                        n2404 = local write "EVENT LOG"(w3469) -> ()
                      }
                      frame #16 {
                        n2405 = Wait (ms)(milliseconds to wait=u32 50) -> ()  [unwired: 1 out]
                      }
                      frame #17 {
                        n2406 = local read "USER ID"() -> (w3472:string)
                        n2407 = Concatenate Strings("Operator ID :" ("Content"), w3472) -> (w3474:string)
                        n2408 = local read "EVENT LOG"() -> (w3476:string)
                        n2409 = call "Event Log.vi"("Content"=w3474, "EVENT LOG"=w3476) -> ("EVENT LOG"=w3475:string)  [unwired: 8 in, 1 out]
                        n2410 = local write "EVENT LOG"(w3475) -> ()
